vi "TrackColor.vi"(3 "Debug":bool, 4 "Track":bool, 5 "Mono Image In 2":T1, 6 "Color Image In":T1) -> (1 "Particles":i32, 2 "ColorImage Out":T1)   [LabVIEW 2017]
uses:
  <vilib>/vision/Image Controls.llb/IMAQ Image.ctl
  <vilib>/vision/NI_Vision_Development_Module.lvlib
panel:
  in  "Blue or Luma Range":cluster{"Lower value":i32, "Upper value":i32}={"Lower value"=0, "Upper value"=255}
  in  "Green or Sat Range":cluster{"Lower value":i32, "Upper value":i32}={"Lower value"=0, "Upper value"=255}
  in  "Red or Hue Range":cluster{"Lower value":i32, "Upper value":i32}={"Lower value"=0, "Upper value"=255}
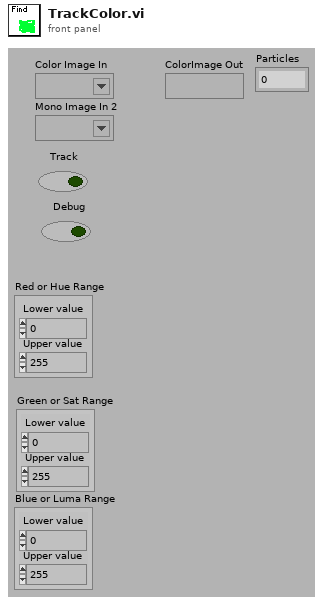
[diagram p1: front panel]
types:
  T1 = typedef "IMAQ Image.ctl" = refnum<image>
  T2 = cluster{"Global Rectangle":i32[], "Contours":cluster{"ID":enum32{"External", "Internal"}, "Type":u32, "Coordinates":i32[]}[]}
  T3 = typedef "IMAQ Rectangle" = cluster{"Left":i32, "Top":i32, "Right":i32, "Bottom":i32, "Rotation":dbl}
  T4 = typedef "ROI Descriptor" = cluster{"Global Rectangle":i32[], "Contours":cluster{"ID":enum32{"External", "Internal"}, "Type":u32, "Coordinates":i32[]}[]}
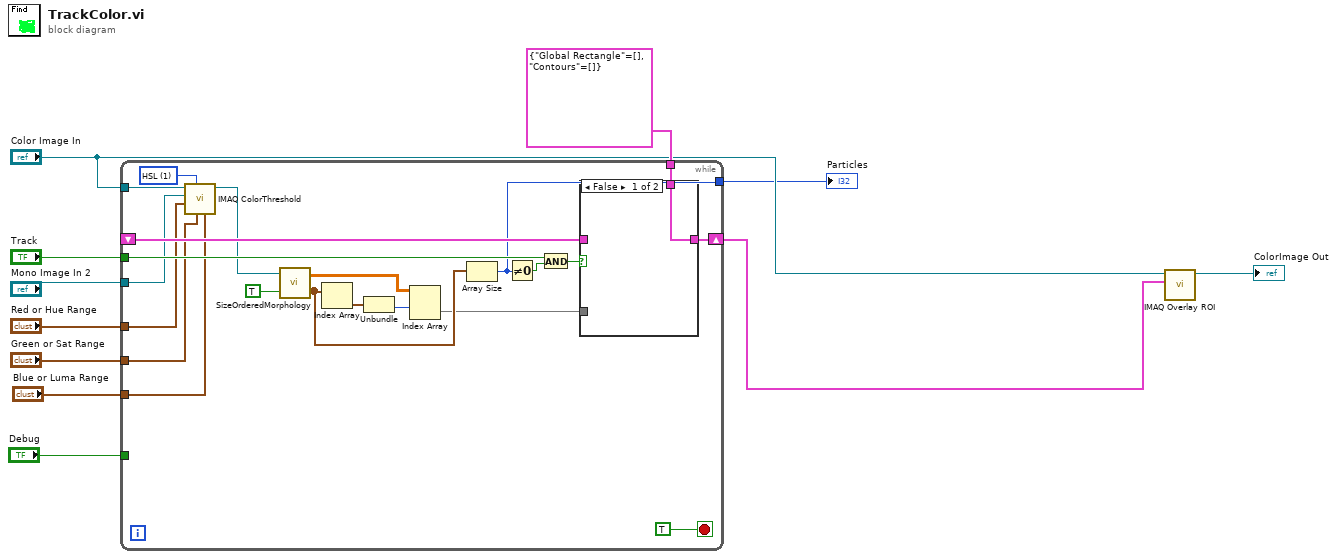
[diagram p0: block diagram]
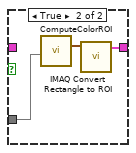
[diagram p2: hidden frame]
diagram:
  n1 = while {
    tunnel: "Mono Image In 2" -> [w24]
    shift-right: [w31] -> w7
    shift-left: _ -> [w26]
    tunnel: "Track" -> [w32]
    tunnel: T2 {"Global Rectangle"=[], "Contours"=[]} ("ROI Descriptor") -> [w30]
    tunnel: "Debug" -> [_]
    tunnel: "Color Image In" -> [w25]
    tunnel: "Red or Hue Range" -> [w23]
    tunnel: "Green or Sat Range" -> [w22]
    tunnel: "Blue or Luma Range" -> [w21]
    tunnel: [w12] -> w1
    stop <- TRUE stop-if-true
    w20 = u16 1 items=["RGB", "HSL", "HSV", "HSI"] ("Color Mode")
    n2 = call "IMAQ ColorThreshold"("Blue or Luma or Val or Inten Range"=w21, "Green or Sat Range"=w22, "Color Mode"=w20, "Red or Hue Range"=w23, "Image Dst"=w24, "Image Src"=w25) -> ("Image Dst Out"=w19:T1)  [unwired: 4 in, 1 out]
    n3 = call <vilib>:"SizeOrderedMorphology.vi"("Green"=TRUE, "Image Dst Out"=w19) -> ("Sort Array"=w14:cluster{"Numeric":dbl, i32}[], "Particle Measurements (Pixels)"=w15:dbl[][])
    n4 = Index Array(array=w14) -> (element=w17:cluster{"Numeric":dbl, i32})  [unwired: 1 in]
    n5 = Unbundle(w17) -> (w16:i32)  [unwired: 1 out]
    n6 = Index Array(array=w15, index (row)=w16) -> (element=w13:dbl[])  [unwired: 1 in]
    n7 = Array Size(array=w14) -> (size(s)=w12:i32)
    n8 = Not Equal To 0?(x=w12) -> (x != 0?=w27:bool)
    n9 = And(x=w32, y=w27) -> (x .and. y?=w28:bool)
    n10 = case shown="False" w28 {
      tunnel: w26 -> [_ _]
      tunnel: [w33 w36] -> w31
      tunnel: w30 -> [w33 _]
      tunnel: w13 -> [_ w35]
      frame False {
      }
      frame True {
        n11 = call <vilib>:"ComputeColorROI.vi"("Array"=w35) -> ("Rectangle"=w34:T3)
        n12 = call "IMAQ Convert Rectangle to ROI"("Rectangle"=w34) -> ("ROI Descriptor"=w36:T4)  [unwired: 8 in, 1 out]
      }
    }
  }
  "Particles" <- w1
  n13 = call "IMAQ Overlay ROI"("ROI Descriptor"=w7, "Image"="Color Image In") -> ("Image Out"=→"ColorImage Out":T1)  [unwired: 8 in, 1 out]
